vi "EstimateTargettingInformation.vi"(0 "Robot X (in)":dbl, 1 "Robot Y (in)":dbl) -> (2 "Estimated Distance to Target (in)":dbl, 3 "Estimated Heading to Target (deg)":dbl)   [LabVIEW 2019]
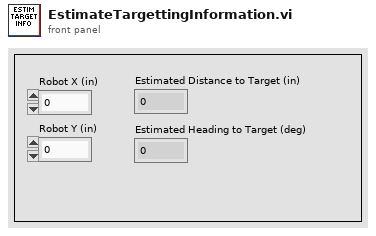
[diagram p1: front panel]
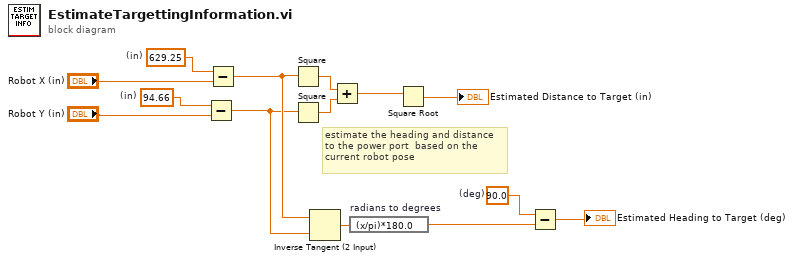
[diagram p0: block diagram]
diagram:
  w5 = 90.0  # (deg)
  w8 = 94.66  # (in)
  w10 = 629.25  # (in)
  # "estimate the heading and distance\nto the power port  based on the\ncurrent robot pose"
  n1 = Subtract(x=w8, y="Robot Y (in)") -> (x-y=w6:dbl)
  n2 = Subtract(x=w10, y="Robot X (in)") -> (x-y=w7:dbl)
  n3 = Square(x=w7) -> (x^2=w14:dbl)
  n4 = Square(x=w6) -> (x^2=w13:dbl)
  n5 = Inverse Tangent (2 Input)(1:w6, 2:w7) -> (0:w3:dbl)
  n6 = Add(x=w14, y=w13) -> (x+y=w12:dbl)
  n7 = expression code="(x/pi)*180.0" "radians to degrees"(w3) -> (w2:dbl)
  n8 = Square Root(x=w12) -> (sqrt(x)=→"Estimated Distance to Target (in)":dbl)
  n9 = Subtract(x=w5, y=w2) -> (x-y=→"Estimated Heading to Target (deg)":dbl)
